vi "PopulateFRT.vi"(11 "Path":path=path "") -> (3 "Array":string[](array[string]))   [LabVIEW 2014]
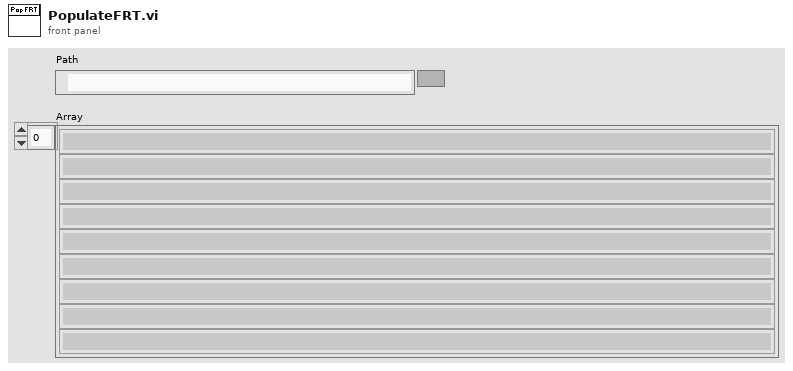
[diagram p1: front panel]
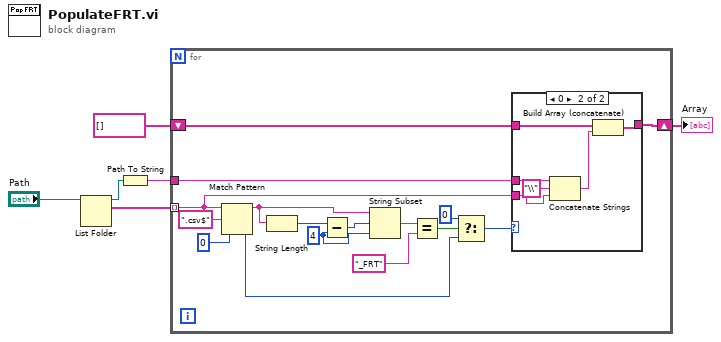
[diagram p0: block diagram]
diagram:
  n1 = List Folder(path="Path") -> (path out=w4:path, filenames=w6:string[])  [unwired: 3 in, 2 out]
  n2 = Path To String(path=w4) -> (string=w3:string)
  n3 = for {
    tunnel: w6 -> [w20] mode=indexing
    tunnel: w3 -> [w19]
    shift-right: [w18] -> w1
    shift-left: string[] [] -> [w17]
    w14 = 4 ("y")
    n4 = Match Pattern(string=w20, regular expression=".csv$", offset (0)=0) -> (before substring=w7:string, offset past match=w10:i32)  [unwired: 2 out]
    n5 = String Length(string=w7) -> (length=w16:i32)
    n6 = Subtract(x=w16, y=w14) -> (x-y=w15:i32)
    n7 = String Subset(string=w7, offset (0)=w15, length (rest)=w14) -> (substring=w13:string)
    n8 = Equal?(x=w13, y="_FRT") -> (x = y?=w11:bool)
    n9 = Select(t=0, s=w11, f=w10) -> (s? t:f=w8:i32)
    n10 = case shown="0" w8 {
      tunnel: w20 -> [_ w24]
      tunnel: w19 -> [_ w29]
      tunnel: [w23 w26] -> w18
      tunnel: w17 -> [w23 w28]
      frame Default {
      }
      frame 0 {
        n11 = Concatenate Strings(w29, "\\" ("string"), w24) -> (w27:string)
        n12 = Build Array (concatenate)(w28, w27) -> (w26:string[])
      }
    }
  }
  "Array" <- w1
